vi "Initialize CAD.vi"(8 "error in (no error)":errorcluster) -> (0 "error out":errorcluster, 1 "Success":bool)   [LabVIEW 2015, in "AguaClara Library.lvlib"]
uses:
  AguaClara Library.lvlib
  AutoCAD cmds.ctl
  Word cmd.ctl
  Folders.ctl
  Mathcad Prime cmds.ctl
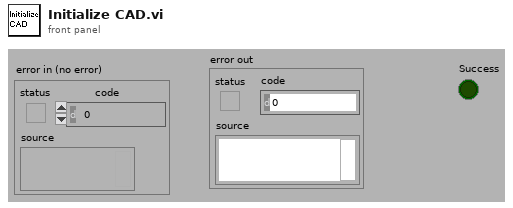
[diagram p1: front panel]
types:
  T1 = typedef "Folders.ctl" = enum16{"DesignTool", "RequestedDesigns", "CompletedDesigns"}
  T2 = typedef "Mathcad Prime cmds.ctl" = enum16{"Open Mathcad", "Open Worksheet", "Send Inputs", "Read Results", "Quit Mathcad"}
  T3 = typedef "AguaClara Library.lvlib/AutoCAD cmds.ctl" = enum16{"Open AutoCAD", "New Document", "Send Command", "Send Command Array", "Close Doc", "Quit"}
  T4 = typedef "AguaClara Library.lvlib/Word cmd.ctl" = enum16{"Initialize", "Load User Inputs", "Update Fields", "Replace Variables", "Save pdf", "Close Word"}
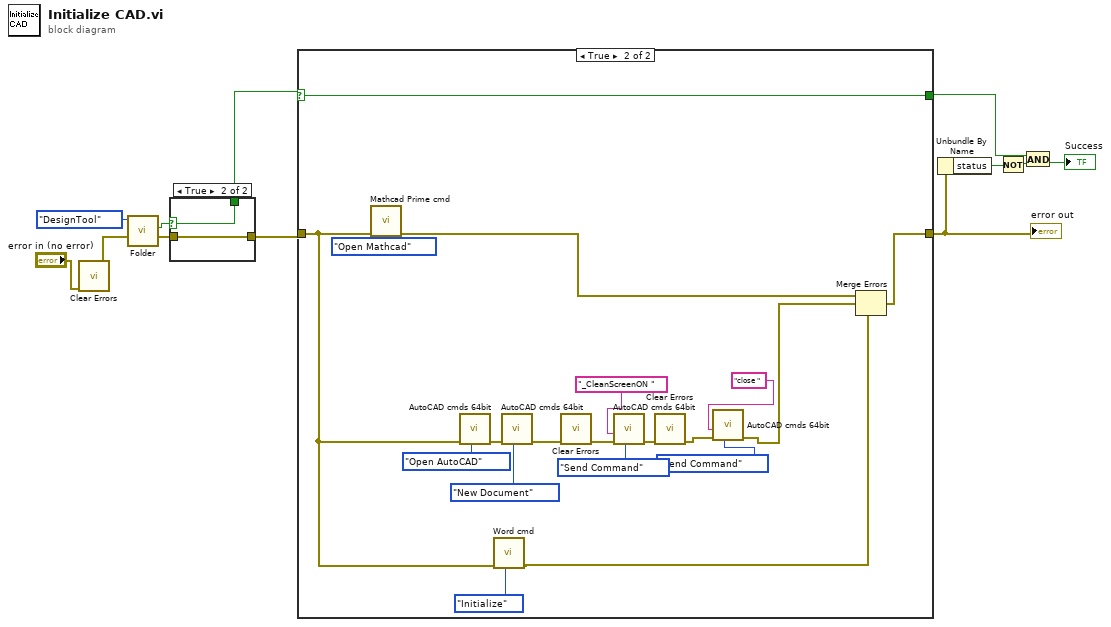
[diagram p0: block diagram]
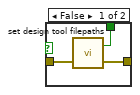
[diagram p2: hidden frame]
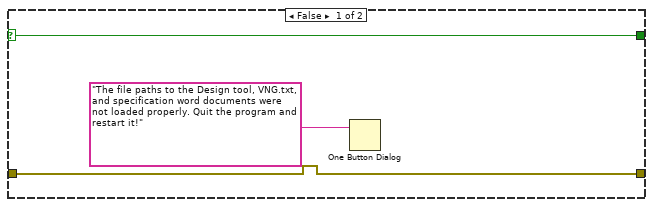
[diagram p3: hidden frame]
diagram:
  n1 = call <vilib>:"Clear Errors.vi"("error in (no error)"="error in (no error)") -> ("error out"=w1:errorcluster)  [unwired: 5 in, 1 out]
  n2 = call "Folder.vi"("Folders"=Folders."DesignTool") -> ("found?"=w2:bool)  [unwired: 9 in, 1 out]
  n3 = case shown="True" w2 {
    selector: w2 -> [_ w16]
    tunnel: [w14 w15] -> w7
    tunnel: [w13 w16] -> w6
    tunnel: w1 -> [w12 w15]
    frame False {
      n4 = call "set design tool filepaths.vi"("error in (no error)"=w12) -> ("error out"=w14:errorcluster, "Success"=w13:bool)  [unwired: 1 in]
    }
    frame True {
    }
  }
  n5 = case shown="True" w6 {
    selector: w6 -> [w19 w37]
    tunnel: [w18 w32] -> w4
    tunnel: [w19 w37] -> w5
    tunnel: w7 -> [w18 w23]
    frame False {
      n6 = One Button Dialog(message="The file paths to the Design tool, VNG.txt, and specification word documents were not loaded properly. Quit the program and restart it!") -> ()  [unwired: 1 in, 1 out]
    }
    frame True {
      n7 = call "Mathcad Prime cmd.vi"("Mathcad Prime cmds"=Mathcad_Prime_cmds."Open Mathcad", "error in (no error)"=w23) -> ("error out"=w21:errorcluster)  [unwired: 7 in, 2 out]
      n8 = call "AutoCAD cmds 64bit.vi"("AutoCAD cmd"=AutoCAD_cmds."Open AutoCAD", "error in (no error)"=w23) -> ("error out"=w31:errorcluster)  [unwired: 7 in, 2 out]
      n9 = call "Word cmd.vi"("Word cmd"=Word_cmd."Initialize", "Error In (no error)"=w23) -> ("error out"=w20:errorcluster)  [unwired: 8 in, 1 out]
      n10 = call "AutoCAD cmds 64bit.vi"("AutoCAD cmd"=AutoCAD_cmds."New Document", "error in (no error)"=w31) -> ("error out"=w30:errorcluster)  [unwired: 7 in, 2 out]
      n11 = call <vilib>:"Clear Errors.vi"("error in (no error)"=w30) -> ("error out"=w28:errorcluster)  [unwired: 5 in, 1 out]
      n12 = call "AutoCAD cmds 64bit.vi"("AutoCAD cmd"=AutoCAD_cmds."Send Command", "error in (no error)"=w28, "Command"="_CleanScreenON ") -> ("error out"=w29:errorcluster)  [unwired: 6 in, 2 out]
      n13 = call <vilib>:"Clear Errors.vi"("error in (no error)"=w29) -> ("error out"=w27:errorcluster)  [unwired: 5 in, 1 out]
      n14 = call "AutoCAD cmds 64bit.vi"("AutoCAD cmd"=AutoCAD_cmds."Send Command", "error in (no error)"=w27, "Command"="close ") -> ("error out"=w25:errorcluster)  [unwired: 6 in, 2 out]
      n15 = Merge Errors(w21, w25, w20) -> (w32:errorcluster)
    }
  }
  "error out" <- w4
  n16 = Unbundle By Name(w4) -> ("status"=w9:bool)
  n17 = Not(x=w9) -> (.not. x?=w10:bool)
  n18 = And(x=w5, y=w10) -> (x .and. y?=→"Success":bool)
